vi "Load SS Implem.vi"(8 "Ball Gatherer State":T1=enum."Positional", 10 "Robot Commands":T3) -> (2 "Load Actuator Values Out":T2)   [LabVIEW 2015]
uses:
  Robot Commands 2016.ctl
  Roller State.ctl
  Load Actuator Values.ctl
  Ball Gatherer State.ctl
  Global Variables/refnum names.vi
  Global Variables/Temp Variables.vi
  Global Variables/Settings.vi
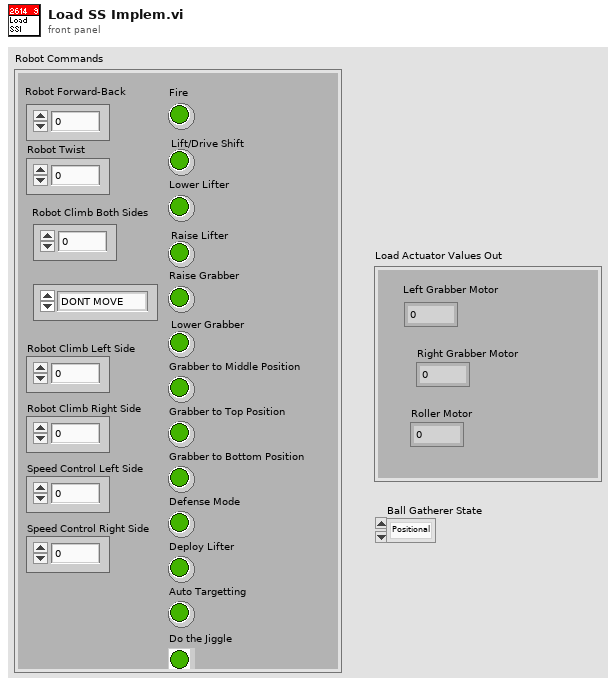
[diagram p1: front panel]
types:
  T1 = typedef "Ball Gatherer State.ctl" = enum16{"Manual", "Positional"}
  T2 = typedef "Load Actuator Values.ctl" = cluster{"Left Grabber Motor":dbl, "Right Grabber Motor":dbl, "Roller Motor":dbl}
  T3 = typedef "Robot Commands 2016.ctl" = cluster{"Robot Forward-Back":dbl, "Robot Twist":dbl, "Fire":bool, "Lift/Drive Shift":bool, "Raise Lifter":bool, "Raise Grabber":bool, "Lower Grabber":bool, "Roller":T4, "Robot Climb Both Sides":dbl, "Grabber to Middle Position":bool, "Grabber to Top Position":bool, "Grabber to Bottom Position":bool, "Robot Climb Left Side":dbl, "Robot Climb Right Side":dbl, "Speed Control Left Side":dbl, "Speed Control Right Side":dbl, "Lower Lifter":bool, "Defense Mode":bool, "Deploy Lifter":bool, "Auto Targetting":bool, "Do the Jiggle":bool}
  T4 = typedef "Roller State.ctl" = enum16{"DONT MOVE", "Intake", "Outtake"}
  T5 = typedef "WPI_MotorControlDeviceRef.ctl" = cluster{"DeviceStatus":errorcluster, "Type":T6, "PWM":cluster{"PWM Channel":T7, "DeadBand":T8}, "CAN":cluster{"Device Number":u8, "Control Mode":T9, "Semaphore":T10, "Max Vout":dbl, "TalonSRX Control Mode":T11}, "Invert":bool}
  T6 = typedef "WPI_MotorControlType.ctl" = enum16{"PWM", "CAN", "CANTalonSRX"}
  T7 = typedef "FPGA_DIOPWMChannel.ctl" = enum8{"PWM 0", "PWM 1", "PWM 2", "PWM 3", "PWM 4", "PWM 5", "PWM 6", "PWM 7", "PWM 8", "PWM 9", "PWM MXP 0", "PWM MXP 1", "PWM MXP 2", "PWM MXP 3", "PWM MXP 4", "PWM MXP 5", "PWM MXP 6", "PWM MXP 7", "PWM MXP 8", "PWM MXP 9", "Invalid"}
  T8 = typedef "WPI_PWMDeadband.ctl" = cluster{"Name":string, "maxPositivePwm":i32, "minPositivePwm":i32, "centerPwm":i32, "maxNegativePwm":i32, "minNegativePwm":i32, "angularRange":u16}
  T9 = typedef "WPI_CANJaguar_ControlMode.ctl" = enum8{"Percent VBus", "Current", "Speed", "Position", "Voltage"}
  T10 = typedef "Semaphore RefNum" = refnum<k1>
  T11 = typedef "WPI_CANTalonSRX_APIControlMode.ctl" = enum8{"Percent VBus", "Speed", "Position", "Slave", "Unchanged / Invalid", "Voltage Compensation", "Current", "Motion Profile"}
  T12 = typedef "WPI_CANTalonSRX_GlobalStatus.ctl" = cluster{"Applied Throttle":dbl, "Module Enabled":bool, "CAN Error":errorcluster, "Closed Loop Error":dbl, "Forward Limit Switch Closed":bool, "Reverse Limit Switch Closed":bool, "Sensor Position":dbl, "Sensor Velocity":dbl, "Current":dbl, "Sticky Fault - Over Temp":bool, "Sticky Fault - Under Voltage":bool, "Sticky Fault - Forward Limit":bool, "Sticky Fault - Reverse Limit":bool, "Sticky Fault - Forward Soft Limit":bool, "Sticky Fault - Reverse Soft Limit":bool, "Brake is Enabled":bool, "Encoder Position":dbl, "Encoder Velocity":dbl, "Encoder Index Count":dbl, "Encoder A Pin State":bool, "Encoder B Pin State":bool, "Encoder Index Pin State":bool, "Analog In":dbl, "Analog In Velocity":dbl, "Temperature (C)":dbl, "Battery Voltage":dbl, "Control 5 Is Supported":bool, "Current Profile Slot Select":dbl, "Pos Div 8":bool, "Vel Div 4":bool, "Pulse Width Position":i32, "Pulse Width Velocity":i32, "Pulse Width Rise To Rise (us)":i32, "Pulse Width Rise To Fall (us)":i32, "Mot Prof Active Is Under Run":bool, "Mot Prof Active Has Under Run":bool, "Mot Prof Active Is Last":bool, "Mot Prof Active Velocity Only":bool, "Mot Prof Active Is Valid":bool, "Mot Prof Buffer Is Full":bool, "Mot Prof Active Profile Slot Select":i32, "Mot Prof NextID":i32, "Mot Prof Count":i32, "Mot Prof Active Velocity":dbl, "Mot Prof Active Position":dbl, "Mot Prof Output Enable":i32}
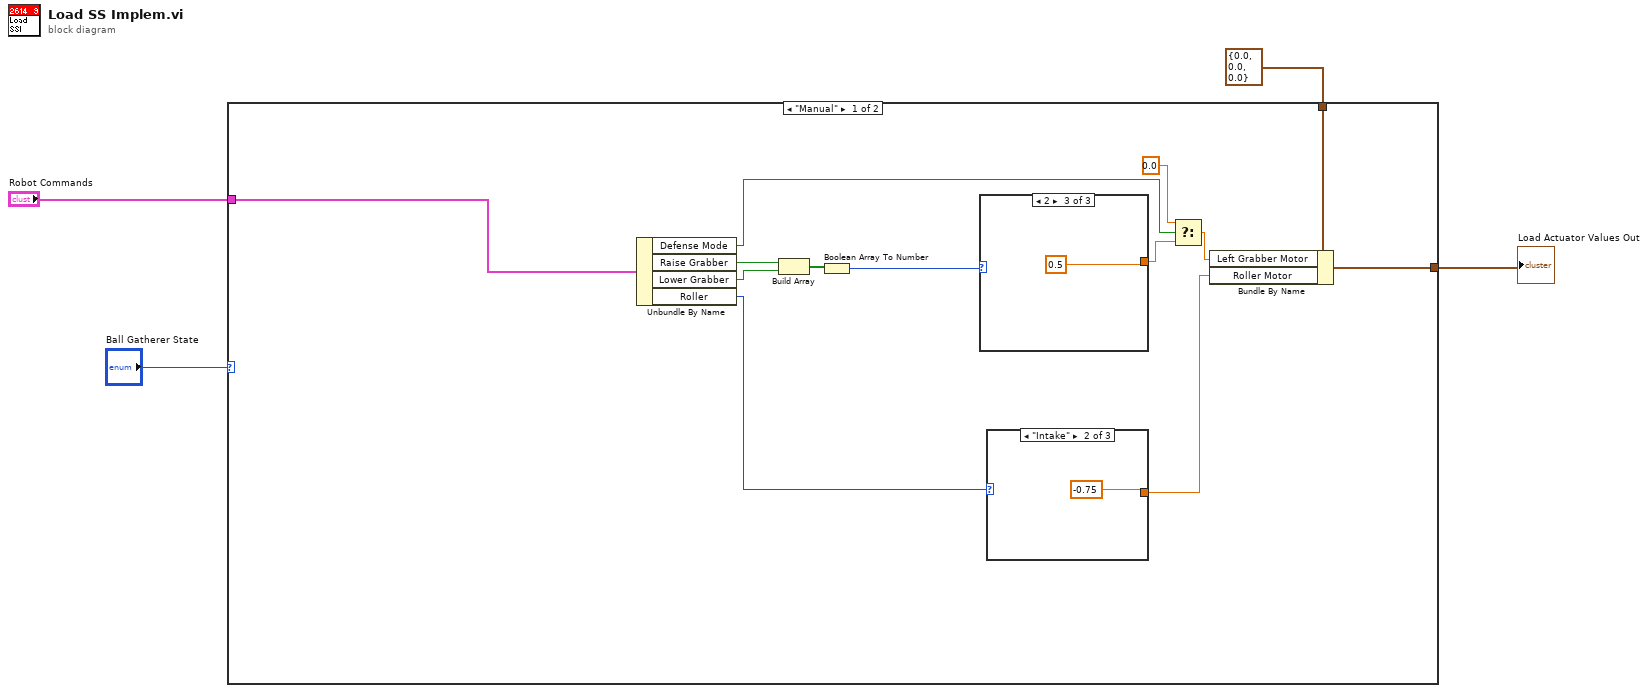
[diagram p0: block diagram]
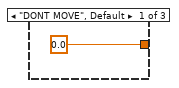
[diagram p2: hidden frame]
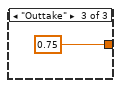
[diagram p3: hidden frame]
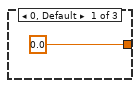
[diagram p4: hidden frame]
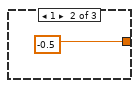
[diagram p5: hidden frame]
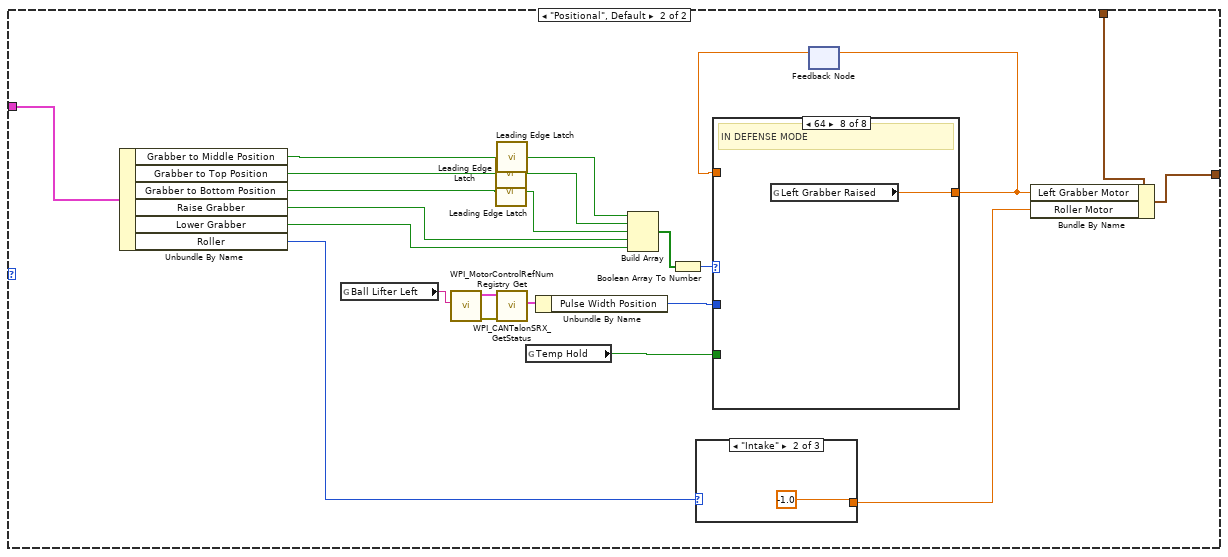
[diagram p6: hidden frame]
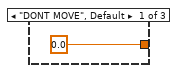
[diagram p7: hidden frame]
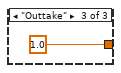
[diagram p8: hidden frame]
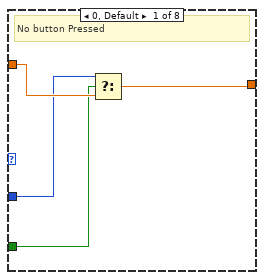
[diagram p9: hidden frame]
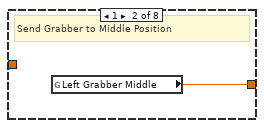
[diagram p10: hidden frame]
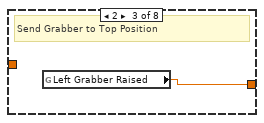
[diagram p11: hidden frame]
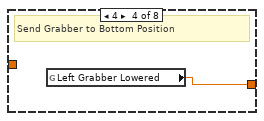
[diagram p12: hidden frame]
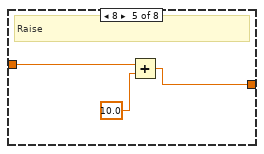
[diagram p13: hidden frame]
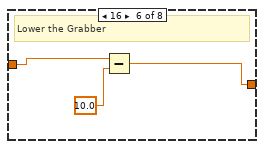
[diagram p14: hidden frame]
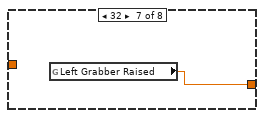
[diagram p15: hidden frame]
diagram:
  n1 = case shown="\"Manual\"" "Ball Gatherer State" {
    tunnel: "Robot Commands" -> [w17 w44]
    tunnel: [w9 w43] -> w2
    tunnel: T2 {"Left Grabber Motor"=0.0, "Right Grabber Motor"=0.0, "Roller Motor"=0.0} ("Load Actuator Values Out 2") -> [w16 w42]
    frame "Manual" {
      n2 = Unbundle By Name(w17) -> ("Defense Mode"=w8:bool, "Raise Grabber"=w15:bool, "Lower Grabber"=w14:bool, "Roller"=w11:T4)
      n3 = Build Array(w15, w14) -> (w13:bool[])
      n4 = Boolean Array To Number(Boolean array=w13) -> (number=w12:u32)
      n5 = case shown="2" w12 {
        tunnel: [0.0 -0.5 0.5] -> w7
        frame 0, Default {
        }
        frame 1 {
        }
        frame 2 {
        }
      }
      n6 = case shown="\"Intake\"" w11 {
        tunnel: [0.0 -0.75 0.75] -> w10
        frame "DONT MOVE", Default {
        }
        frame "Intake" {
        }
        frame "Outtake" {
        }
      }
      n7 = Select(t=0.0, s=w8, f=w7) -> (s? t:f=w6:dbl)
      n8 = Bundle By Name(cluster=w16, "Left Grabber Motor"=w6, "Roller Motor"=w10) -> (w9:T2)
    }
    frame "Positional", Default {
      n9 = Unbundle By Name(w44) -> ("Grabber to Middle Position"=w33:bool, "Grabber to Top Position"=w32:bool, "Grabber to Bottom Position"=w31:bool, "Raise Grabber"=w35:bool, "Lower Grabber"=w26:bool, "Roller"=w41:T4)
      n10 = global read "refnum names.vi" "Ball Lifter Left"() -> (w39:string)
      n11 = call <vilib>:"WPI_MotorControlRefNum Registry Get.vi"("refnum name"=w39) -> ("error out"=w38:errorcluster, "MotorControlDevRef"=w37:T5)  [unwired: 9 in]
      n12 = call "Leading Edge Latch.vi"("Input"=w32) -> ("Output"=w29:bool)
      n13 = call "Leading Edge Latch.vi"("Input"=w31) -> ("Output"=w28:bool)
      n14 = call "Leading Edge Latch.vi"("Input"=w33) -> ("Output"=w30:bool)
      n15 = call <vilib>:"WPI_CANTalonSRX_GetStatus.vi"("error in (no error)"=w38, "CAN Talon SRX Ref"=w37) -> ("Talon SRX Status"=w36:T12)  [unwired: 7 in, 2 out]
      n16 = global read "Temp Variables.vi" "Temp Hold"() -> (w24:bool)
      n17 = Unbundle By Name(w36) -> ("Pulse Width Position"=w25:i32)
      n18 = Build Array(w30, w29, w28, w35, w26) -> (w45:bool[])
      n19 = Boolean Array To Number(Boolean array=w45) -> (number=w46:u32)
      n20 = case shown="\"Intake\"" w41 {
        tunnel: [0.0 -1.0 1.0] -> w40
        frame "DONT MOVE", Default {
        }
        frame "Intake" {
        }
        frame "Outtake" {
        }
      }
      n21 = feedback #1() -> (w34:dbl)  [unwired: 1 in]
      n22 = case shown="64" w46 {
        tunnel: [w52 w54 w55 w56 w57 w60 w63 w64] -> w27
        tunnel: w34 -> [w53 _ _ _ w58 w61 _ _]
        tunnel: w25 -> [w51 _ _ _ _ _ _ _]
        tunnel: w24 -> [w50 _ _ _ _ _ _ _]
        frame 0, Default {
          # "No button Pressed"
          n23 = Select(t=w51, s=w50, f=w53) -> (s? t:f=w52:dbl)
        }
        frame 1 {
          # "Send Grabber to Middle Position"
          n24 = global read "Settings.vi" "Left Grabber Middle"() -> (w54:dbl)
        }
        frame 2 {
          # "Send Grabber to Top Position"
          n25 = global read "Settings.vi" "Left Grabber Raised"() -> (w55:dbl)
        }
        frame 4 {
          # "Send Grabber to Bottom Position"
          n26 = global read "Settings.vi" "Left Grabber Lowered"() -> (w56:dbl)
        }
        frame 8 {
          # "Raise"
          n27 = Add(x=w58, y=10.0 ("x")) -> (x+y=w57:dbl)
        }
        frame 16 {
          # "Lower the Grabber"
          n28 = Subtract(x=w61, y=10.0 ("x")) -> (x-y=w60:dbl)
        }
        frame 32 {
          n29 = global read "Settings.vi" "Left Grabber Raised"() -> (w63:dbl)
        }
        frame 64 {
          # "IN DEFENSE MODE"
          n30 = global read "Settings.vi" "Left Grabber Raised"() -> (w64:dbl)
        }
      }
      n31 = feedback-in #1(w27) -> ()
      n32 = Bundle By Name(cluster=w42, "Left Grabber Motor"=w27, "Roller Motor"=w40) -> (w43:T2)
    }
  }
  "Load Actuator Values Out" <- w2
